vi "Create.vi"(10 "Status":T1) -> (3 "Sequencing Status Value out":refnum<class "Sequencing Status Value.lvclass">)   [LabVIEW 2020, in "VolatusSeq.lvlib" / "Sequencing Status Value.lvclass"]
uses:
  Sequencing Status Value.lvclass
  Sequencing Status.ctl
  Sequence Status Extended.ctl
  Sequence Status.ctl
  Sequence Time.ctl
  Sequencing Status Value.lvclass/Sequencing Status Value.ctl
  VolatusSeq.lvlib
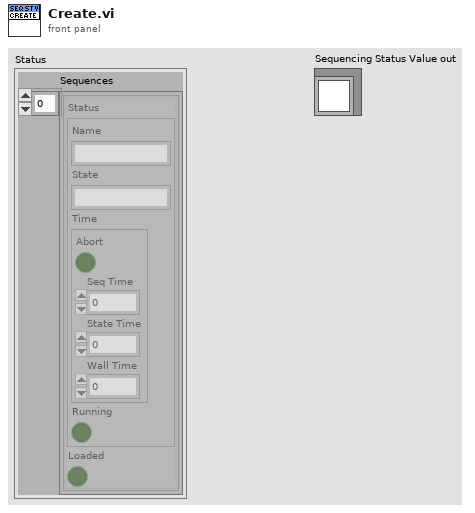
[diagram p1: front panel]
types:
  T1 = typedef "VolatusSeq.lvlib/Sequencing Status.ctl" = cluster{"Sequences":T2[]}
  T2 = typedef "VolatusSeq.lvlib/Sequence Status Extended.ctl" = cluster{"Status":T3, "Loaded":bool}
  T3 = typedef "VolatusSeq.lvlib/Sequence Status.ctl" = cluster{"Name":string, "State":string, "Time":T4, "Running":bool}
  T4 = typedef "VolatusSeq.lvlib/Sequence Time.ctl" = cluster{"Abort":bool, "Seq Time":dbl, "State Time":dbl, "Wall Time":dbl}
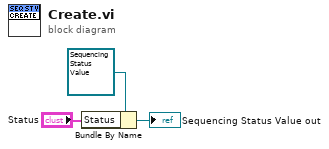
[diagram p0: block diagram]
diagram:
  n1 = Bundle By Name(cluster=refnum<class "Sequencing Status Value.lvclass"> refnum ("Sequencing Status Value in"), "Status"="Status") -> (→"Sequencing Status Value out":refnum<class "Sequencing Status Value.lvclass">)
